vi "Remove SubVI.vi"() -> ()   [LabVIEW 2017]
panel:
  in  "Remove SubVI":bool
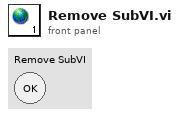
[diagram p1: front panel]
diagram:
